vi "Enum Shunt to Gain.vi"(1 "Shunt Resistor":T1 items=["Open", "50 Ohms", "500 Ohms", "5k Ohms", "50k Ohms", "10M Ohm"]) -> (0 "Gain (V/A)":dbl)   [LabVIEW 2019, in "KH7008.lvlib"]
uses:
  KH7008.lvlib
  typedefs/shunt--ring.ctl
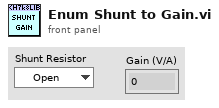
[diagram p1: front panel]
types:
  T1 = typedef "KH7008.lvlib/shunt--ring.ctl" = u32
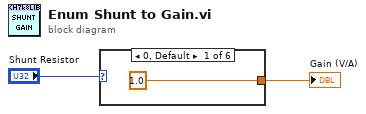
[diagram p0: block diagram]
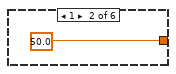
[diagram p2: hidden frame]
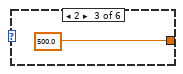
[diagram p3: hidden frame]
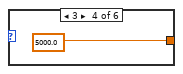
[diagram p4: hidden frame]
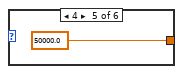
[diagram p5: hidden frame]
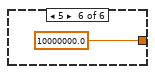
[diagram p6: hidden frame]
diagram:
  n1 = case shown="0, Default" "Shunt Resistor" {
    tunnel: [1.0 ("y") 50.0 ("y") 500.0 ("y") 5000.0 ("y") 50000.0 ("y") 10000000.0 ("y")] -> w1
    frame 0, Default {
    }
    frame 1 {
    }
    frame 2 {
    }
    frame 3 {
    }
    frame 4 {
    }
    frame 5 {
    }
  }
  "Gain (V/A)" <- w1
